vi "Proceed Image.vi"(8 "error in (no error)":errorcluster, 10 "Image":T1, 11 "IMAQ Display in":refnum<class "HIJ Vision Display.lvclass">) -> (0 "error out":errorcluster, 3 "HIJ Vision Display out":refnum<class "HIJ Vision Display.lvclass">)   [LabVIEW 2020, in "HIJ Vision Display.lvlib" / "HIJ Vision Display.lvclass"]
doc: "Das VI wird bei jedem neuen Bild aufgerufen. \nEs ist eine Statische Aktion des Aktors. Damit soll sichergestellt sein,\ndass Pre Process.vi vor dem Analyze.vi aufgerufen wird. \n\nPre Process zeitg Standarausgeben wie Ziel- und Schwerpunktkreuz. \nAlte Overlays werden gelöscht. Die Kindklassen wie z.B. IMAQdx Display können Pre Process.vi\nerweitern und z.B. ein Hintergrundbild abziehen. Nach Preprocessing wird\ndas Bild angezeigt. Bis hierher ist die Operation synchron. Es wird davon ausgegangen, dass\nPreprocessing schnell genug ist, und vor dem nachkommenden Bild abgeschlossen wird.\n\nDas eigentliche Auswerten des Bildes wird in Analyze Actor (AA) ausgelagert. Analyze.vi schickt\neine asynchrone Nachricht an Analyze Actor. Wenn der AA fertig ist, schickt er eine Nachricht \nmit Ergebnissen zurück. Je nach Komplexität der Auswertung, kann es passieren, dass Display \nActor beriets ein neues Bild anzeigt. Diese Situation kann anhand der Bildnummernvergleiches\nerkannt werden."
uses:
  HIJ Vision Display.lvclass
  <vilib>/vision/Image Controls.llb/IMAQ Image.ctl
  HIJ Vision Display.lvclass/HIJ Vision Display.ctl
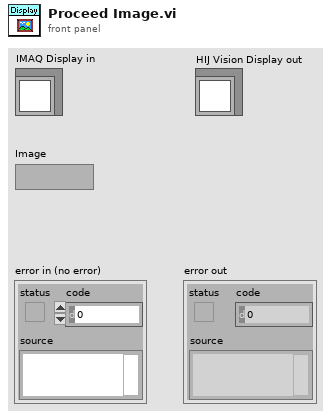
[diagram p1: front panel]
types:
  T1 = typedef "IMAQ Image.ctl" = refnum<image>
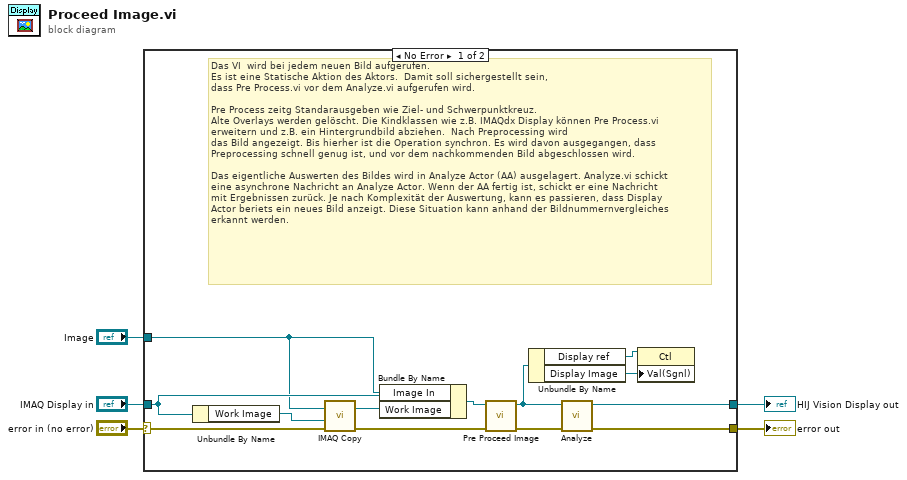
[diagram p0: block diagram]
diagram:
  n1 = case shown="No Error" "error in (no error)" {
    selector: "error in (no error)" -> [w16 w20]
    tunnel: [w17 w20] -> w4
    tunnel: "IMAQ Display in" -> [w18 w19]
    tunnel: "Image" -> [w6 _]
    tunnel: [w15 w19] -> w1
    frame No Error {
      # "Das VI  wird bei jedem neuen Bild aufgerufen. \nEs ist eine Statische Aktion des Aktors.  Damit soll sichergestellt sein,\ndass Pre Process.vi vor dem Analyze.vi aufgerufen wird. \n\nPre Process zeitg Standarausgeben wie Ziel- und Schwerpunktkreuz. \nAlte Overlays werden gelöscht. Die Kindklassen wie z.B. IMAQdx Display können Pre Process.vi\nerweitern und z.B. ein Hintergrundbild abziehen.  Nach Preprocessing wird\ndas Bild angezeigt. Bis hierher ist die Operation synchron. Es wird davon ausgegangen, dass\nPreprocessing schnell genug ist, und vor dem nachkommenden Bild abgeschlossen wird.\n\nDas eigentliche Auswerten des Bildes wird in Analyze Actor (AA) ausgelagert. Analyze.vi schickt\neine asynchrone Nachricht an Analyze Actor. Wenn der AA fertig ist, schickt er eine Nachricht \nmit Ergebnissen zurück. Je nach Komplexität der Auswertung, kann es passieren, dass Display \nActor beriets ein neues Bild anzeigt. Diese Situation kann anhand der Bildnummernvergleiches\nerkannt werden."
      n2 = Unbundle By Name(w18) -> ("Work Image"=w10:T1)
      n3 = call "IMAQ Copy"("error in (no error)"=w16, "Image Dst"=w10, "Image Src"=w6) -> ("error out"=w12:errorcluster, "Image Dst Out"=w7:T1)  [unwired: 3 in]
      n4 = Bundle By Name(cluster=w18, "Image In"=w6, "Work Image"=w7) -> (w8:refnum<class "HIJ Vision Display.lvclass">)
      n5 = call-dynamic "Pre Proceed Image.vi"("error in (no error)"=w12, "Display in"=w8) -> ("error out"=w11:errorcluster, "Display out"=w13:refnum<class "HIJ Vision Display.lvclass">)  [unwired: 8 in]
      n6 = Unbundle By Name(w13) -> ("Display ref"=w14:refnum<vi>, "Display Image"=w9:T1)
      n7 = call-dynamic "Analyze.vi"("error in (no error)"=w11, "HIJ Vision Display in"=w13) -> ("error out"=w17:errorcluster, "HIJ Vision Display out"=w15:refnum<class "HIJ Vision Display.lvclass">)  [unwired: 8 in]
      n8 = property class="Ctl"(reference=w14, "Val(Sgnl)"=w9) -> ()  [unwired: 1 in, 2 out]
    }
    frame Error {
    }
  }
  "error out" <- w4
  "HIJ Vision Display out" <- w1
